vi "Fin_GlobalData.vi"() -> ()   [LabVIEW 2015]
panel:
  in  "RasnilStiffRef":path=path "/home/atlas/Desktop/LWDAQ/Data_stiffback/Results20170823085343.txt"
  in  "RasnilTableRef":path=path "/home/atlas/Desktop/LWDAQ/Data_table/Results20170823085217.txt"
  out "xlos5":dbl=106.92
  out "xlos4":dbl=83.16
  out "xlos2":dbl=35.64
  out "xlos3":dbl=59.4
  out "xlos1":dbl=11.88
  out "ylos04":dbl=47.52
  out "ylos06":dbl=71.28
  out "sin-phi":dbl=-0.00239
  out "cos-phi":dbl=0.99999712
  out "phi":dbl=-0.0024
  out "y-offset":dbl=60.0
  out "x-offset":dbl=24.0
  out "d-param-x-surveyor":dbl=27.888
  out "d-param-y-surveyor":dbl=76.253
  in  "DryRun":string
  in  "Stage":string
  in  "PanelName":string
  in  "strip":string="Eta"
  in  "quota":string="Table"
  in  "Password":string="alcione2"
  in  "programma":string
  in  "operator":string="nobody"
  # "s"
  # "(Table or Stiffback)"
  # "(Stereo or Eta)"
  # "Stiffback/Table"
  # "Full/Empty"
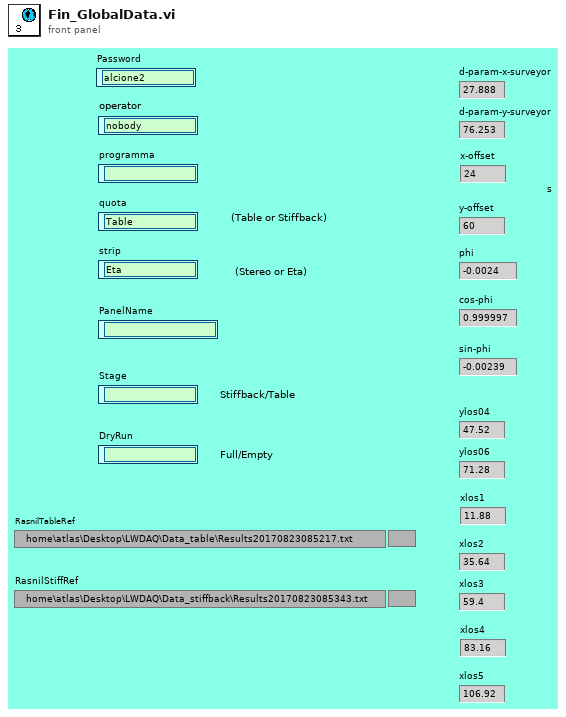
[diagram p1: front panel]
diagram:
